vi "test Close Standard Input.vi"(8 "error in":errorcluster) -> (0 "error out":errorcluster)   [LabVIEW 2020, in "serenial.io-ase.test.lvlib"]
uses:
  serenial.io-ase.test.lvlib
  serenial.io-ase/ase/Standard Input State.ctl
  serenial.io-ase/ase/ase.lvclass/ase.ctl
  serenial.io-ase/ase/Merge Call Library Errors.vi
  serenial.io-ase/ase/Error Invalid ASE Handle.vi
  serenial.io-ase/ase/Error Internal Library Implementation Error.vi
  <vilib>/Utility/file.llb/Application Directory.vi
  <vilib>/Utility/error.llb/Error Cluster From Error Code.vi
  <vilib>/addons/_JKI Toolkits/Caraya/classes/Assert/Assert Not Error.vi
  <vilib>/addons/_JKI Toolkits/Caraya/classes/Assert/Assert Equal Value and Type_Variant.vi
  serenial.io-ase/ase/Wait on Call.vi
  <vilib>/addons/_JKI Toolkits/Caraya/classes/Assert/Assert.lvclass
  <vilib>/addons/_JKI Toolkits/Caraya/classes/Test/Test.lvclass
  serenial.io-ase/ase/ase.lvclass
  serenial.io-ase/ase/Start Call (Exe-Args).vi
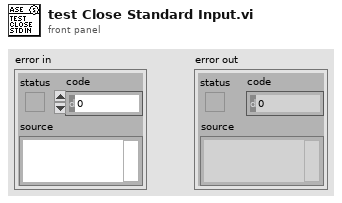
[diagram p1: front panel]
types:
  T1 = typedef "serenial.io-ase.lvlib/ase.lvclass/Standard Input State.ctl" = enum16{"Open/Closing", "Closed"}
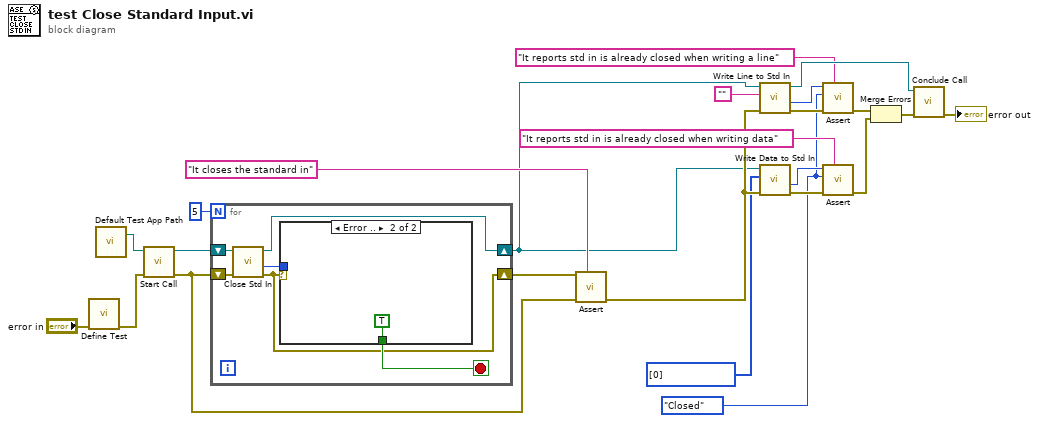
[diagram p0: block diagram]
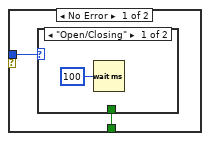
[diagram p2: hidden frame]
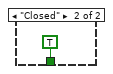
[diagram p3: hidden frame]
diagram:
  w4 = Standard_Input_State."Closed" ("State")
  n1 = call <vilib>:"Define Test.vi"("error in (no error)"="error in") -> ("error out"=w21:errorcluster)  [unwired: 10 in]
  n2 = call "Default Test App Path.vi"() -> ("Exe Path With Extention"=w1:path)  [unwired: 2 in, 1 out]
  n3 = call-poly "Start Call.vi"("error in"=w21, "Executable Path"=w1) -> ("error out"=w22:errorcluster, "New ASE Handle"=w11:refnum<class "ase.lvclass">)  [unwired: 8 in]
  n4 = for {
    N: 5 -> [_]
    shift-right: [w25] -> w23
    shift-left: w22 -> [w30]
    shift-right: [w28] -> w6
    shift-left: w11 -> [w29]
    stop <- w26 stop-if-true
    n5 = call "Close Std In.vi"("error in"=w30, "ASE Handle"=w29) -> ("error out"=w25:errorcluster, "State"=w27:T1, "ASE Handle Duplicate"=w28:refnum<class "ase.lvclass">)  [unwired: 7 in]
    n6 = case shown="Error .." w25 {
      tunnel: w27 -> [w32 _]
      tunnel: [w31 TRUE] -> w26
      frame No Error {
        n7 = case shown="\"Open/Closing\"" w32 {
          tunnel: [_ TRUE] -> w31
          frame "Open/Closing" {
            n8 = Wait (ms)(milliseconds to wait=u32 100) -> ()  [unwired: 1 out]
          }
          frame "Closed" {
          }
        }
      }
      frame Error {
      }
    }
  }
  n9 = call-poly <vilib>:"Assert.vi"("Label"="It closes the standard in", "error in (no error)"=w22, "Not Error?"=w23) -> ("error out"=w17:errorcluster)  [unwired: 8 in]
  n10 = call "Write Line to Std In .vi"("error in"=w17, "Input"="" ("Empty String Constant"), "ASE Handle"=w6) -> ("error out"=w7:errorcluster, "State"=w3:T1, "ASE Handle Duplicate"=w10:refnum<class "ase.lvclass">)  [unwired: 6 in]
  n11 = call "Write Data to Std In.vi"("error in"=w17, "Data"=u8[] [0], "ASE Handle"=w6) -> ("error out"=w15:errorcluster, "State"=w5:T1)  [unwired: 6 in, 1 out]
  n12 = call-poly <vilib>:"Assert.vi"("Label"="It reports std in is already closed when writing a line", "error in (no error)"=w7, "Y"=w4, "X"=w3) -> ("error out"=w19:errorcluster)  [unwired: 7 in]
  n13 = call-poly <vilib>:"Assert.vi"("Label"="It reports std in is already closed when writing data", "error in (no error)"=w15, "Y"=w4, "X"=w5) -> ("error out"=w13:errorcluster)  [unwired: 7 in]
  n14 = Merge Errors(w19, w13) -> (w14:errorcluster)
  n15 = call "Conclude Call.vi"("error in"=w14, "ASE Handle"=w10) -> ("error out"=→"error out":errorcluster)  [unwired: 7 in, 2 out]
